vi "create missles.vi"(6 "key in":T1(ring), 7 "current missles":cluster{i32, i32, i32}[](array[cluster]), 9 "orinetation":i32, 10 "column":i32, 11 "row":i32) -> (2 "number of missles":i32, 3 "missles position out":cluster{i32, i32, i32}[](array[cluster]))   [LabVIEW 2019]
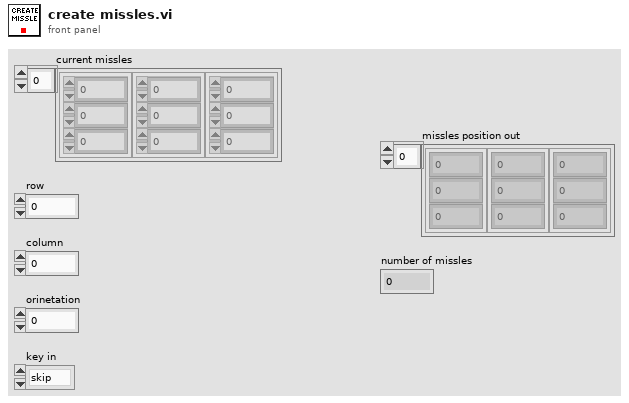
[diagram p1: front panel]
types:
  T1 = enum16{"skip", "prawo", "lewo", "ruch", "strzal"}
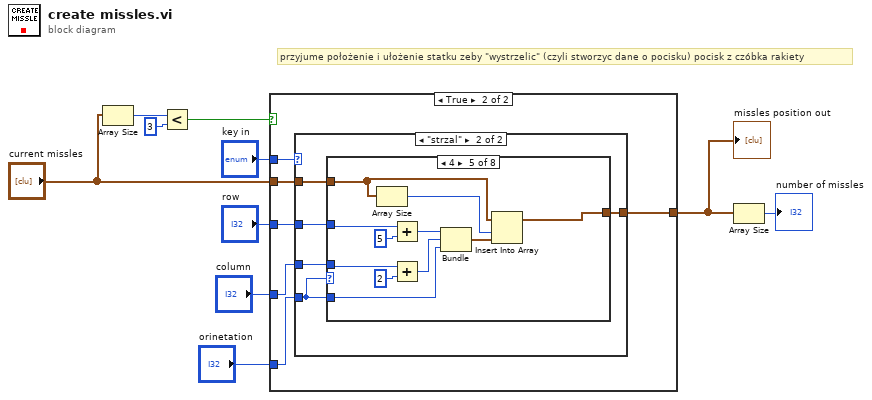
[diagram p0: block diagram]
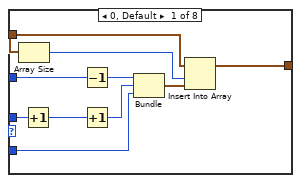
[diagram p4: hidden frame]
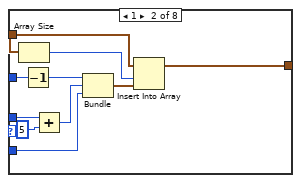
[diagram p5: hidden frame]
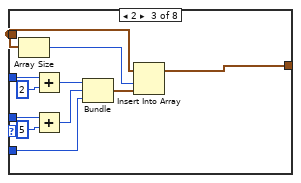
[diagram p6: hidden frame]
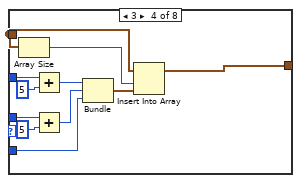
[diagram p7: hidden frame]
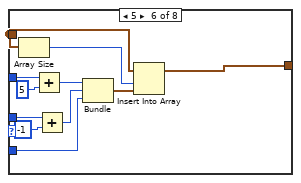
[diagram p8: hidden frame]
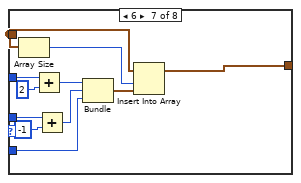
[diagram p9: hidden frame]
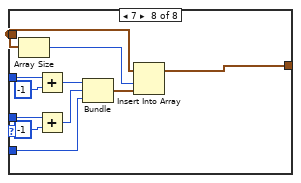
[diagram p10: hidden frame]
diagram:
  # "przyjume położenie i ułożenie statku zeby \"wystrzelic\" (czyli stworzyc dane o pocisku) pocisk z czóbka rakiety"
  n1 = Array Size(array="current missles") -> (size(s)=w3:i32)
  n2 = Less?(x=w3, y=3) -> (x < y?=w9:bool)
  n3 = case shown="True" w9 {
    tunnel: "key in" -> [_ w17]
    tunnel: "orinetation" -> [_ w16]
    tunnel: "column" -> [_ w15]
    tunnel: "row" -> [_ w14]
    tunnel: "current missles" -> [w11 w13]
    tunnel: [w11 w12] -> w2
    frame False {
    }
    frame True {
      n4 = case shown="\"strzal\"" w17 {
        tunnel: w16 -> [_ w21]
        tunnel: w15 -> [_ w23]
        tunnel: w14 -> [_ w22]
        tunnel: w13 -> [w18 w20]
        tunnel: [w18 w19] -> w12
        frame "skip", Default {
        }
        frame "strzal" {
          n5 = case shown="4" w21 {
            tunnel: w23 -> [w33 w36 w46 w57 w68 w79 w90 w101]
            tunnel: w22 -> [w31 w38 w49 w60 w71 w82 w93 w104]
            tunnel: w21 -> [w30 w40 w50 w61 w72 w83 w94 w105]
            tunnel: w20 -> [w26 w39 w51 w62 w73 w84 w95 w106]
            tunnel: [w24 w41 w52 w63 w74 w85 w96 w107] -> w19
            frame 0, Default {
              n6 = Array Size(array=w26) -> (size(s)=w25:i32)
              n7 = Increment(x=w33) -> (x+1=w32:i32)
              n8 = Decrement(x=w31) -> (x-1=w28:i32)
              n9 = Increment(x=w32) -> (x+1=w29:i32)
              n10 = Bundle(w28, w29, "orinetation"=w30) -> (w27:cluster{i32, i32, "orinetation":i32})  [unwired: 1 in]
              n11 = Insert Into Array(array=w26, index=w25, new element=w27) -> (w24:cluster{i32, i32, i32}[])
            }
            frame 1 {
              n12 = Array Size(array=w39) -> (size(s)=w42:i32)
              n13 = Decrement(x=w38) -> (x-1=w37:i32)
              n14 = Add(x=w36, y=5) -> (x+y=w34:i32)
              n15 = Bundle(w37, w34, "orinetation"=w40) -> (w43:cluster{i32, i32, "orinetation":i32})  [unwired: 1 in]
              n16 = Insert Into Array(array=w39, index=w42, new element=w43) -> (w41:cluster{i32, i32, i32}[])
            }
            frame 2 {
              n17 = Array Size(array=w51) -> (size(s)=w53:i32)
              n18 = Add(x=w49, y=2) -> (x+y=w47:i32)
              n19 = Add(x=w46, y=5) -> (x+y=w44:i32)
              n20 = Bundle(w47, w44, "orinetation"=w50) -> (w54:cluster{i32, i32, "orinetation":i32})  [unwired: 1 in]
              n21 = Insert Into Array(array=w51, index=w53, new element=w54) -> (w52:cluster{i32, i32, i32}[])
            }
            frame 3 {
              n22 = Array Size(array=w62) -> (size(s)=w64:i32)
              n23 = Add(x=w60, y=5) -> (x+y=w58:i32)
              n24 = Add(x=w57, y=5) -> (x+y=w55:i32)
              n25 = Bundle(w58, w55, "orinetation"=w61) -> (w65:cluster{i32, i32, "orinetation":i32})  [unwired: 1 in]
              n26 = Insert Into Array(array=w62, index=w64, new element=w65) -> (w63:cluster{i32, i32, i32}[])
            }
            frame 4 {
              n27 = Array Size(array=w73) -> (size(s)=w75:i32)
              n28 = Add(x=w71, y=5) -> (x+y=w69:i32)
              n29 = Add(x=w68, y=2) -> (x+y=w66:i32)
              n30 = Bundle(w69, w66, "orinetation"=w72) -> (w76:cluster{i32, i32, "orinetation":i32})  [unwired: 1 in]
              n31 = Insert Into Array(array=w73, index=w75, new element=w76) -> (w74:cluster{i32, i32, i32}[])
            }
            frame 5 {
              n32 = Array Size(array=w84) -> (size(s)=w86:i32)
              n33 = Add(x=w82, y=5) -> (x+y=w80:i32)
              n34 = Add(x=w79, y=-1) -> (x+y=w77:i32)
              n35 = Bundle(w80, w77, "orinetation"=w83) -> (w87:cluster{i32, i32, "orinetation":i32})  [unwired: 1 in]
              n36 = Insert Into Array(array=w84, index=w86, new element=w87) -> (w85:cluster{i32, i32, i32}[])
            }
            frame 6 {
              n37 = Array Size(array=w95) -> (size(s)=w97:i32)
              n38 = Add(x=w93, y=2) -> (x+y=w91:i32)
              n39 = Add(x=w90, y=-1) -> (x+y=w88:i32)
              n40 = Bundle(w91, w88, "orinetation"=w94) -> (w98:cluster{i32, i32, "orinetation":i32})  [unwired: 1 in]
              n41 = Insert Into Array(array=w95, index=w97, new element=w98) -> (w96:cluster{i32, i32, i32}[])
            }
            frame 7 {
              n42 = Array Size(array=w106) -> (size(s)=w108:i32)
              n43 = Add(x=w104, y=-1) -> (x+y=w102:i32)
              n44 = Add(x=w101, y=-1) -> (x+y=w99:i32)
              n45 = Bundle(w102, w99, "orinetation"=w105) -> (w109:cluster{i32, i32, "orinetation":i32})  [unwired: 1 in]
              n46 = Insert Into Array(array=w106, index=w108, new element=w109) -> (w107:cluster{i32, i32, i32}[])
            }
          }
        }
      }
    }
  }
  "missles position out" <- w2
  n47 = Array Size(array=w2) -> (size(s)=→"number of missles":i32)
